vi "MEMR-Initialize Stimuli.vi"(0 "Data folder":path, 5 "Params":T31, 7 "AO in":T1 {"noiseChan"."Filter"."Stages"."IIR Filter"."Forward Coefficients" format="%.4f"; "noiseChan"."Filter"."Stages"."IIR Filter"."Reverse Coefficients" format="%.4f"}, 11 "error in (no error)":errorcluster) -> (8 "AO out":T1 {"noiseChan"."Filter"."Stages"."IIR Filter"."Forward Coefficients" format="%.4f"; "noiseChan"."Filter"."Stages"."IIR Filter"."Reverse Coefficients" format="%.4f"}, 15 "error out":errorcluster)   [LabVIEW 2020]
uses:
  Typedefs/MEMR-Params.ctl
  Typedefs/MEMR-Probe.ctl
  Typedefs/MEMR-Elicitor.ctl
  Human Studies/SFM Frontend/LV Source/Typedefs/HSTS-Transducer.ctl
  Typedefs/MEMR-Sequence.ctl
  Typedefs/MEMR-Analysis.ctl
  Typedefs/MEMR-Timing.ctl
  Typedefs/MEMR-AO Data.ctl
  Signal Synthesis VIs/3rd Generation/XControls/Stimulus Channel (G3)/Full Stimulus Channel Data.ctl
  Signal Synthesis VIs/3rd Generation/XControls/Waveform XControls/Waveform (G3)/Waveform Data.ctl
  Signal Synthesis VIs/3rd Generation/Waveform VIs/Waveform Enum (V3).ctl
  Signal Synthesis VIs/3rd Generation/XControls/Waveform XControls/Tone (G3)/Tone.Properties.ctl
  Signal Synthesis VIs/Waveform VIs/Pulse Train VIs/Pulse Train Params.ctl
  Signal Synthesis VIs/Waveform VIs/Pulse Train VIs/Pulse Polarity.ctl
  Signal Synthesis VIs/Waveform VIs/Pulse Train VIs/PT-Continuous State.ctl
  Signal Synthesis VIs/3rd Generation/Waveform VIs/Noise VIs/Noise (G3).ctl
  Signal Synthesis VIs/3rd Generation/Waveform VIs/Noise VIs/Noise (G3).Properties.ctl
  Signal Synthesis VIs/3rd Generation/Waveform VIs/Noise VIs/Noise (G3).Data.ctl
  Signal Synthesis VIs/Waveform VIs/File VIs/StimFile-Params.ctl
  Signal Synthesis VIs/Waveform VIs/FM Sweep VIs/FM Sweep Params.ctl
  Signal Synthesis VIs/Waveform VIs/Chirp Train VIs/Chirp Train.ctl
  Signal Synthesis VIs/Waveform VIs/Chirp Train VIs/Chirp Train Params.ctl
  Signal Synthesis VIs/Waveform VIs/Complex Tone VIs/CT-Params.ctl
  Signal Synthesis VIs/Waveform VIs/Complex Tone VIs/CT-Phase Enum.ctl
  Signal Synthesis VIs/Waveform VIs/Complex Tone VIs/CT-Runtime Data.ctl
  Signal Synthesis VIs/3rd Generation/XControls/Waveform XControls/FM Tone/Data.ctl
  Signal Synthesis VIs/3rd Generation/XControls/Waveform XControls/Vowel/Vowel.Properties.ctl
  Signal Synthesis VIs/3rd Generation/Waveform VIs/Ramp VIs/Ramp.Properties.ctl
  Signal Synthesis VIs/3rd Generation/XControls/Filter (G3)/Filter Data.ctl
  Signal Synthesis VIs/3rd Generation/XControls/Filter (G3)/Filter Type.ctl
  Signal Synthesis VIs/Filter VIs/Filter-Bandwidth Units.ctl
  Signal Synthesis VIs/Controls/Burst XCtl/Burst Data.ctl
  Signal Synthesis VIs/3rd Generation/XControls/Level (G3)/Level Data.ctl
  Signal Synthesis VIs/3rd Generation/XControls/Level (G3)/Level Units (G3).ctl
  Signal Synthesis VIs/3rd Generation/XControls/Advanced Options (G3)/Advanced Options (G3).ctl
  Signal Synthesis VIs/Modulation VIs/SAM VIs/SAM Params.ctl
  Signal Synthesis VIs/3rd Generation/Typedefs/Destination.ctl
  PXI DAQ VIs/DAQ Engine VIs/PXI Globals.vi
  Utility VIs/Math VIs/LinSpace (start-stop-step).vi
  Utility VIs/Math VIs/dB to Linear (1D).vi
  Signal Synthesis VIs/3rd Generation/XControls/Waveform XControls/Tone (G3)/Tone (G3).xctl
  Signal Synthesis VIs/3rd Generation/XControls/Waveform XControls/FM Tone/FM Tone.xctl
  Signal Synthesis VIs/3rd Generation/XControls/Waveform XControls/Vowel/Vowel.xctl
  Signal Synthesis VIs/3rd Generation/XControls/Waveform XControls/Waveform (G3)/Waveform (G3).xctl
  Signal Synthesis VIs/3rd Generation/XControls/Filter (G3)/Filter (G3).xctl
  Signal Synthesis VIs/Controls/Burst XCtl/Burst Control.xctl
  Signal Synthesis VIs/3rd Generation/XControls/Level (G3)/Level (G3).xctl
  Signal Synthesis VIs/3rd Generation/XControls/Advanced Options (G3)/Advanced Options (G3).xctl
  Signal Synthesis VIs/3rd Generation/XControls/Stimulus Channel (G3)/Stimulus Channel (G3).xctl
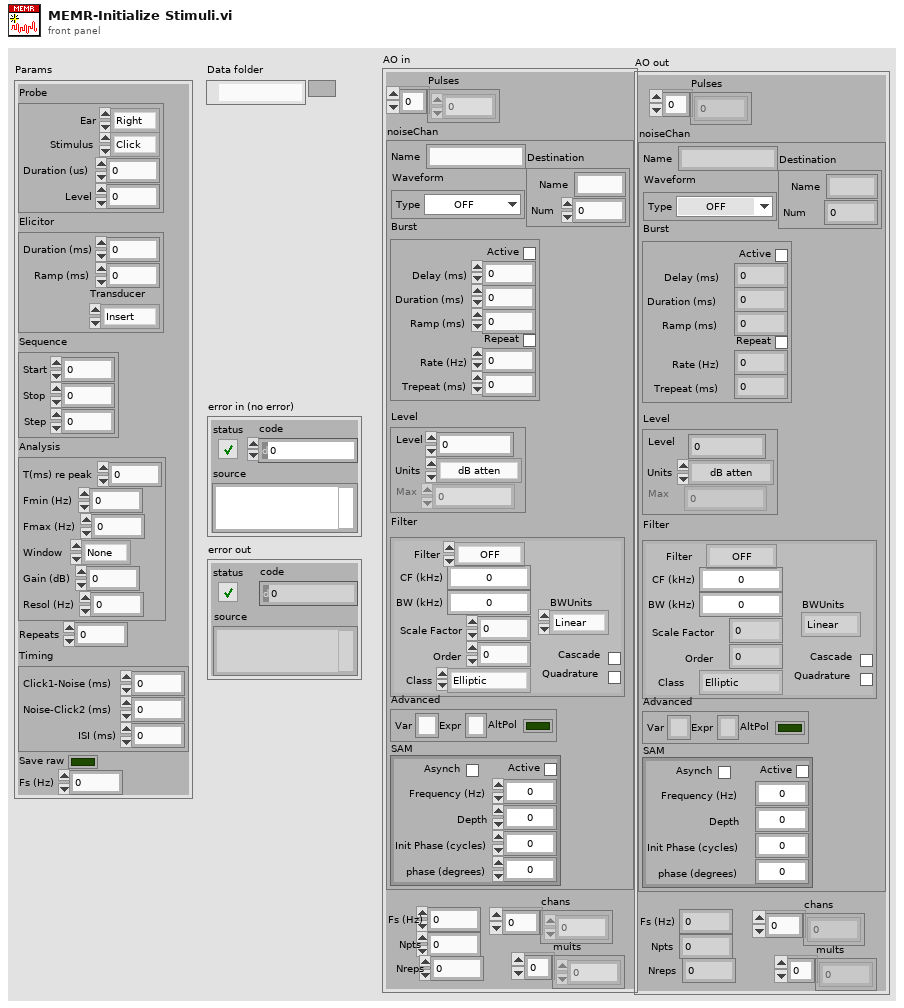
[diagram p1: front panel]
types:
  T1 = typedef "MEMR-AO Data.ctl" = cluster{"Pulses":dbl[], "noiseChan":T2, "Fs (Hz)":dbl, "Npts":i32, "mults":dbl[], "chans":i32[], "Nreps":i32}
  T2 = typedef "Stimulus Channel (G3).xctl/Full Stimulus Channel Data.ctl" = cluster{"Waveform":T3, "Filter":T22, "Burst":T25, "Level":T26, "Name":string, "Advanced":T28, "SAM":T29, "Destination":T30}
  T3 = typedef "Waveform (G3).xctl/Waveform Data.ctl" = cluster{"Type":T4, "Tone":T5, "Pulse Train":T6, "Noise":T9, "File":T12, "FMSweep":T13, "Chirp Train":T14, "Complex Tone":cluster{"Params":T16, "Data":T18}, "FM":T19, "Vowel":T20, "Ramp":T21}
  T4 = typedef "Waveform Enum (V3).ctl" = enum16{"OFF", "Tone", "Noise", "Pulse Train", "File", "FM Sweep", "Chirp Train", "Complex Tone", "FM Tone", "Vowel", "Ramp"}
  T5 = typedef "Tone (G3).xctl/Tone.Properties.ctl" = cluster{"Frequency (kHz)":dbl, "Phase (cycles)":dbl, "Random phase":bool}
  T6 = typedef "Pulse Train Params.ctl" = cluster{"Pulse width (us)":dbl, "Pulse rate (Hz)":dbl, "Gap (ms)":dbl, "Polarity":T7, "PT State":T8, "Asynch":bool}
  T7 = typedef "Pulse Polarity.ctl" = enum16{"POS", "NEG", "POS-NEG", "NEG-POS"}
  T8 = typedef "PT-Continuous State.ctl" = cluster{"Template":dbl[], "Nperiod":i32, "Index":i32, "Pulse Rate (Hz)":dbl, "Phase (cycles)":dbl, "Noff":i32}
  T9 = typedef "Noise (G3).ctl" = cluster{"Properties":T10, "Data":T11}
  T10 = typedef "Noise (G3).Properties.ctl" = cluster{"InvFilt":bool, "Aweight":bool, "Seed":i32, "Tokens":i32, "Brickwall":bool}
  T11 = typedef "Noise (G3).Data.ctl" = cluster{"TokenNum":i32}
  T12 = typedef "StimFile-Params.ctl" = cluster{"Filename":path, "Signal":dbl[], "Channel":i32, "stream":bool, "offset":i32, "nreps":i32, "loops":i32, "Randomize":bool, "order":i32[], "Seed":i32, "Tokens":i32}
  T13 = typedef "FM Sweep Params.ctl" = cluster{"Rate (oct/s)":dbl, "Fmin (Hz)":dbl, "Fmax (Hz)":dbl, "Ramp (ms)":dbl, "Linear":bool}
  T14 = typedef "Chirp Train.ctl" = cluster{"Params":T15, "Data":cluster{"WF":dbl[]}}
  T15 = typedef "Chirp Train Params.ctl" = cluster{"Fmin (kHz)":dbl, "Fmax (kHz)":dbl, "Compensate":bool, "Duration (ms)":dbl}
  T16 = typedef "CT-Params.ctl" = cluster{"F0 (Hz)":dbl, "Band":cluster{"Flow (Hz)":dbl, "Fhigh (Hz)":dbl}, "Phase":T17, "Min F0 (Hz)":dbl, "Max F0 (Hz)":dbl, "ContinRandPhase":bool, "Max peak factor":dbl, "Max mod depth":dbl, "MinHarmNum":i32, "MaxHarmNum":i32, "Level Mode":enum16{"per component", "overall rms"}, "% jitter":dbl}
  T17 = typedef "CT-Phase Enum.ctl" = enum16{"Cosine", "Random", "Alternating"}
  T18 = typedef "CT-Runtime Data.ctl" = cluster{"Ncomp":i32, "MinHarm":i32, "Phase":dbl[], "Amplitude":dbl[], "Npts/frame":i32, "Last F0":dbl, "Fmin":dbl, "Fmax":dbl, "Lslope":dbl, "randphase":bool, "overall rms":bool, "fmult":dbl[], "jittered":bool}
  T19 = typedef "FM Tone.xctl/Data.ctl" = cluster{"Carrier (kHz)":dbl, "ModRate (Hz)":dbl, "Depth (Hz)":dbl, "Phase (cycles)":dbl}
  T20 = typedef "Vowel.xctl/Vowel.Properties.ctl" = cluster{"Freqs":string, "Set level":enum16{"Total", "Per component"}, "Freq":dbl[], "weights":dbl[]}
  T21 = typedef "Ramp.Properties.ctl" = cluster{"Duration (ms)":dbl}
  T22 = typedef "Filter (G3).xctl/Filter Data.ctl" = cluster{"Type":T23, "CF (kHz)":dbl, "BW (kHz)":dbl, "Cascade":bool, "Quadrature":bool, "Scale Factor":dbl, "Stages":cluster{"IIR Filter":cluster{"filter structure":enum32{"IIR 2nd Order", "IIR 4th Order"}, "Reverse Coefficients":dbl[], "Forward Coefficients":dbl[]}, "State":dbl[]}[], "Class":enum16{"Elliptic", "Butterworth"}, "Order":i32, "BWUnits":T24}
  T23 = typedef "Filter (G3).xctl/Filter Type.ctl" = enum16{"OFF", "Lowpass", "Highpass", "Bandpass", "Bandstop"}
  T24 = typedef "Filter-Bandwidth Units.ctl" = enum16{"Linear", "Octaves", "Min-Max"}
  T25 = typedef "Burst Control.xctl/Burst Data.ctl" = cluster{"Active":bool, "Delay (ms)":dbl, "Duration (ms)":dbl, "Ramp (ms)":dbl, "Rate (Hz)":dbl, "Trepeat (ms)":dbl, "Repeat":bool}
  T26 = typedef "Level (G3).xctl/Level Data.ctl" = cluster{"Level":dbl, "Units":T27, "Max":dbl, "Data":cluster{"Multiplier":dbl, "Cal File":path, "Cal":cluster{"Freq (Hz)":dbl[], "Mag (dB SPL)":dbl[], "Phase (deg)":dbl[]}, "audiogram":path}}
  T27 = typedef "Level (G3).xctl/Level Units (G3).ctl" = enum16{"dB atten", "dB SPL", "dB re 1 Vrms", "dB V/Hz½", "mW", "dB HL", "Volts", "dB mW"}
  T28 = typedef "Advanced Options (G3).xctl/Advanced Options (G3).ctl" = cluster{"AltPol":bool, "Var":string, "Expr":string}
  T29 = typedef "SAM Params.ctl" = cluster{"Active":bool, "Frequency (Hz)":dbl, "Depth":dbl, "Init Phase (cycles)":dbl, "phase (degrees)":dbl, "Asynch":bool}
  T30 = typedef "Destination.ctl" = cluster{"Name":string, "Num":i32}
  T31 = typedef "MEMR-Params.ctl" = cluster{"Probe":T32, "Elicitor":T33, "Sequence":T35, "Analysis":T36, "Repeats":i32, "Timing":T37, "Save raw":bool, "Fs (Hz)":dbl}
  T32 = typedef "MEMR-Probe.ctl" = cluster{"Ear":enum16{"Right", "Left"}, "Stimulus":enum16{"Click", "Chirp"}, "Duration (us)":dbl, "Level":dbl}
  T33 = typedef "MEMR-Elicitor.ctl" = cluster{"Duration (ms)":dbl, "Ramp (ms)":dbl, "Transducer":T34}
  T34 = typedef "HSTS-Transducer.ctl" = enum16{"Insert", "TDH-39", "HD300", "ER-10X"}
  T35 = typedef "MEMR-Sequence.ctl" = cluster{"Start":dbl, "Stop":dbl, "Step":dbl}
  T36 = typedef "MEMR-Analysis.ctl" = cluster{"T(ms) re peak":dbl, "Fmin (Hz)":dbl, "Fmax (Hz)":dbl, "Window":enum16{"None", "Hanning", "Hamming"}, "Gain (dB)":dbl, "Resol (Hz)":dbl}
  T37 = typedef "MEMR-Timing.ctl" = cluster{"Click1-Noise (ms)":dbl, "Noise-Click2 (ms)":dbl, "ISI (ms)":dbl}
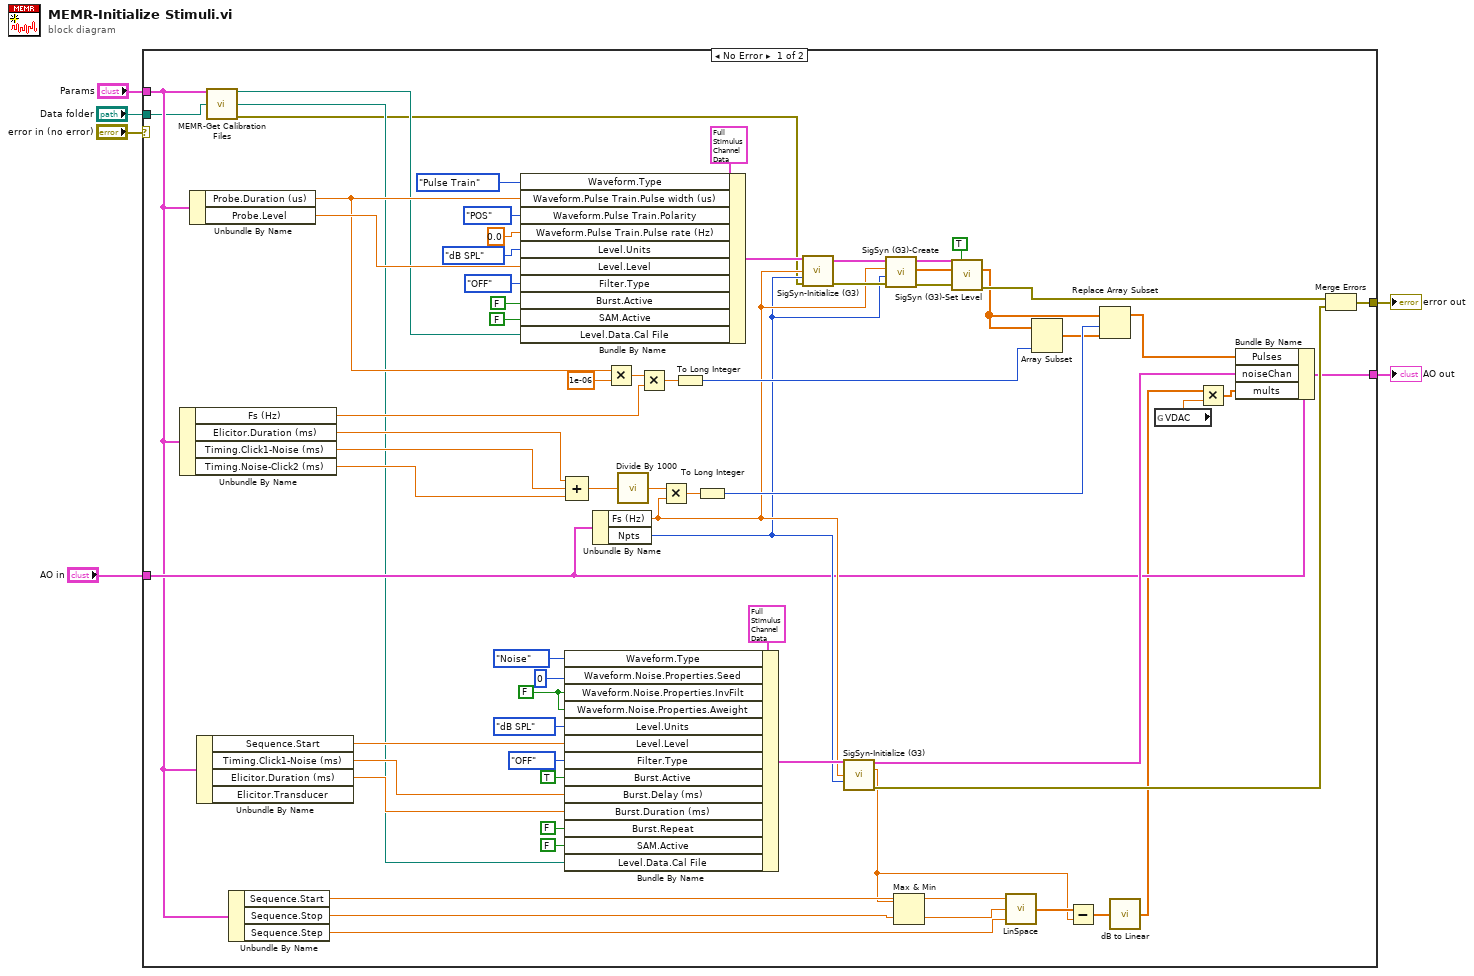
[diagram p0: block diagram]
diagram:
  n1 = case shown="No Error" "error in (no error)" {
    selector: "error in (no error)" -> [_ w75]
    tunnel: "Data folder" -> [w8 _]
    tunnel: [w37 w75] -> w4
    tunnel: "Params" -> [w12 _]
    tunnel: [w25 _] -> w2
    tunnel: "AO in" -> [w22 _]
    frame No Error {
      w48 = FALSE ("Waveform.Noise.Properties.InvFilt")
      n2 = Unbundle By Name(w12) -> ("Fs (Hz)"=w34:dbl, "Elicitor.Duration (ms)"=w62:dbl, "Timing.Click1-Noise (ms)"=w61:dbl, "Timing.Noise-Click2 (ms)"=w60:dbl)
      n3 = Unbundle By Name(w12) -> ("Probe.Duration (us)"=w56:dbl, "Probe.Level"=w69:dbl)
      n4 = Unbundle By Name(w12) -> ("Sequence.Start"=w46:dbl, "Timing.Click1-Noise (ms)"=w43:dbl, "Elicitor.Duration (ms)"=w42:dbl)  [unwired: 1 out]
      n5 = call "MEMR-Get Calibration Files.vi"("Params"=w12, "Data Folder"=w8) -> ("Probe"=w11:path, "Elicitor"=w10:path, "error out"=w9:errorcluster)  [unwired: 11 in]
      n6 = Unbundle By Name(w12) -> ("Sequence.Start"=w32:dbl, "Sequence.Stop"=w30:dbl, "Sequence.Step"=w31:dbl)
      n7 = Bundle By Name(cluster=T2 {"Waveform"={"Type"=enum."Tone", "Tone"={"Frequency (kHz)"=0.0, "Phase (cycles)"=0.0, "Random phase"=FALSE}, "Pulse Train"={"Pulse width (us)"=0.0, "Pulse rate (Hz)"=0.0, "Gap (ms)"=0.0, "Polarity"=enum."POS", "PT State"={"Template"=[], "Nperiod"=0, "Index"=0, "Pulse Rate (Hz)"=0.0, "Phase (cycles)"=0.0, "Noff"=0}, "Asynch"=FALSE}, "Noise"={"Properties"={"InvFilt"=FALSE, "Aweight"=FALSE, "Seed"=0, "Tokens"=0, "Brickwall"=FALSE}, "Data"={"TokenNum"=0}}, "File"={"Filename"=path "", "Signal"=[], "Channel"=0, "stream"=FALSE, "offset"=0, "nreps"=0, "loops"=0, "Randomize"=FALSE, "order"=[], "Seed"=0, "Tokens"=0}, "FMSweep"={"Rate (oct/s)"=0.0, "Fmin (Hz)"=0.0, "Fmax (Hz)"=0.0, "Ramp (ms)"=0.0, "Linear"=FALSE}, "Chirp Train"={"Params"={"Fmin (kHz)"=4.0, "Fmax (kHz)"=64.0, "Compensate"=FALSE, "Duration (ms)"=2.0}, "Data"={"WF"=[]}}, "Complex Tone"={"Params"={"F0 (Hz)"=0.0, "Band"={"Flow (Hz)"=0.0, "Fhigh (Hz)"=0.0}, "Phase"=enum."Cosine", "Min F0 (Hz)"=0.0, "Max F0 (Hz)"=0.0, "ContinRandPhase"=FALSE, "Max peak factor"=inf, "Max mod depth"=2.0, "MinHarmNum"=0, "MaxHarmNum"=0, "Level Mode"=enum."per component", "% jitter"=0.0}, "Data"={"Ncomp"=0, "MinHarm"=0, "Phase"=[], "Amplitude"=[], "Npts/frame"=0, "Last F0"=0.0, "Fmin"=0.0, "Fmax"=0.0, "Lslope"=0.0, "randphase"=FALSE, "overall rms"=FALSE, "fmult"=[], "jittered"=FALSE}}, "FM"={"Carrier (kHz)"=0.0, "ModRate (Hz)"=0.0, "Depth (Hz)"=0.0, "Phase (cycles)"=0.0}, "Vowel"={"Freqs"="", "Set level"=enum."Total", "Freq"=[], "weights"=[]}, "Ramp"={"Duration (ms)"=0.0}}, "Filter"={"Type"=enum."Lowpass", "CF (kHz)"=0.0, "BW (kHz)"=0.0, "Cascade"=FALSE, "Quadrature"=FALSE, "Scale Factor"=0.0, "Stages"=[], "Class"=enum."Elliptic", "Order"=0, "BWUnits"=enum."Linear"}, "Burst"={"Active"=FALSE, "Delay (ms)"=0.0, "Duration (ms)"=0.0, "Ramp (ms)"=0.0, "Rate (Hz)"=0.0, "Trepeat (ms)"=0.0, "Repeat"=FALSE}, "Level"={"Level"=0.0, "Units"=enum."dB atten", "Max"=0.0, "Data"={"Multiplier"=0.0, "Cal File"=path "", "Cal"={"Freq (Hz)"=[], "Mag (dB SPL)"=[], "Phase (deg)"=[]}, "audiogram"=path ""}}, "Name"="", "Advanced"={"AltPol"=FALSE, "Var"="", "Expr"=""}, "SAM"={"Active"=FALSE, "Frequency (Hz)"=0.0, "Depth"=0.0, "Init Phase (cycles)"=0.0, "phase (degrees)"=0.0, "Asynch"=FALSE}, "Destination"={"Name"="", "Num"=0}} ("Stimulus"), "Waveform.Type"=Waveform_Enum_(V3)."Pulse Train", "Waveform.Pulse Train.Pulse width (us)"=w56, "Waveform.Pulse Train.Polarity"=Pulse_Polarity."POS", "Waveform.Pulse Train.Pulse rate (Hz)"=0.0, "Level.Units"=Level_Units_(G3)."dB SPL", "Level.Level"=w69, "Filter.Type"=Filter_Type."OFF", "Burst.Active"=FALSE, "SAM.Active"=FALSE, "Level.Data.Cal File"=w11) -> (w65:T2)
      n8 = Bundle By Name(cluster=T2 {"Waveform"={"Type"=enum."Tone", "Tone"={"Frequency (kHz)"=0.0, "Phase (cycles)"=0.0, "Random phase"=FALSE}, "Pulse Train"={"Pulse width (us)"=0.0, "Pulse rate (Hz)"=0.0, "Gap (ms)"=0.0, "Polarity"=enum."POS", "PT State"={"Template"=[], "Nperiod"=0, "Index"=0, "Pulse Rate (Hz)"=0.0, "Phase (cycles)"=0.0, "Noff"=0}, "Asynch"=FALSE}, "Noise"={"Properties"={"InvFilt"=FALSE, "Aweight"=FALSE, "Seed"=0, "Tokens"=0, "Brickwall"=FALSE}, "Data"={"TokenNum"=0}}, "File"={"Filename"=path "", "Signal"=[], "Channel"=0, "stream"=FALSE, "offset"=0, "nreps"=0, "loops"=0, "Randomize"=FALSE, "order"=[], "Seed"=0, "Tokens"=0}, "FMSweep"={"Rate (oct/s)"=0.0, "Fmin (Hz)"=0.0, "Fmax (Hz)"=0.0, "Ramp (ms)"=0.0, "Linear"=FALSE}, "Chirp Train"={"Params"={"Fmin (kHz)"=4.0, "Fmax (kHz)"=64.0, "Compensate"=FALSE, "Duration (ms)"=2.0}, "Data"={"WF"=[]}}, "Complex Tone"={"Params"={"F0 (Hz)"=0.0, "Band"={"Flow (Hz)"=0.0, "Fhigh (Hz)"=0.0}, "Phase"=enum."Cosine", "Min F0 (Hz)"=0.0, "Max F0 (Hz)"=0.0, "ContinRandPhase"=FALSE, "Max peak factor"=inf, "Max mod depth"=2.0, "MinHarmNum"=0, "MaxHarmNum"=0, "Level Mode"=enum."per component", "% jitter"=0.0}, "Data"={"Ncomp"=0, "MinHarm"=0, "Phase"=[], "Amplitude"=[], "Npts/frame"=0, "Last F0"=0.0, "Fmin"=0.0, "Fmax"=0.0, "Lslope"=0.0, "randphase"=FALSE, "overall rms"=FALSE, "fmult"=[], "jittered"=FALSE}}, "FM"={"Carrier (kHz)"=0.0, "ModRate (Hz)"=0.0, "Depth (Hz)"=0.0, "Phase (cycles)"=0.0}, "Vowel"={"Freqs"="", "Set level"=enum."Total", "Freq"=[], "weights"=[]}, "Ramp"={"Duration (ms)"=0.0}}, "Filter"={"Type"=enum."Lowpass", "CF (kHz)"=0.0, "BW (kHz)"=0.0, "Cascade"=FALSE, "Quadrature"=FALSE, "Scale Factor"=0.0, "Stages"=[], "Class"=enum."Elliptic", "Order"=0, "BWUnits"=enum."Linear"}, "Burst"={"Active"=FALSE, "Delay (ms)"=0.0, "Duration (ms)"=0.0, "Ramp (ms)"=0.0, "Rate (Hz)"=0.0, "Trepeat (ms)"=0.0, "Repeat"=FALSE}, "Level"={"Level"=0.0, "Units"=enum."dB atten", "Max"=0.0, "Data"={"Multiplier"=0.0, "Cal File"=path "", "Cal"={"Freq (Hz)"=[], "Mag (dB SPL)"=[], "Phase (deg)"=[]}, "audiogram"=path ""}}, "Name"="", "Advanced"={"AltPol"=FALSE, "Var"="", "Expr"=""}, "SAM"={"Active"=FALSE, "Frequency (Hz)"=0.0, "Depth"=0.0, "Init Phase (cycles)"=0.0, "phase (degrees)"=0.0, "Asynch"=FALSE}, "Destination"={"Name"="", "Num"=0}} ("Stimulus"), "Waveform.Type"=Waveform_Enum_(V3)."Noise", "Waveform.Noise.Properties.Seed"=0, "Waveform.Noise.Properties.InvFilt"=w48, "Waveform.Noise.Properties.Aweight"=w48, "Level.Units"=Level_Units_(G3)."dB SPL", "Level.Level"=w46, "Filter.Type"=Filter_Type."OFF", "Burst.Active"=TRUE, "Burst.Delay (ms)"=w43, "Burst.Duration (ms)"=w42, "Burst.Repeat"=FALSE, "SAM.Active"=FALSE, "Level.Data.Cal File"=w10) -> (w39:T2)
      n9 = Compound Arithmetic op=ADD(w62, w61, w60) -> (w57:dbl)
      n10 = Unbundle By Name(w22) -> ("Fs (Hz)"=w24:dbl, "Npts"=w23:i32)
      n11 = Multiply(x=w56, y=1e-06) -> (x*y=w53:dbl)
      n12 = call "Divide By 1000.vi"("X"=w57) -> ("X/1000"=w59:dbl)
      n13 = Multiply(x=w53, y=w34) -> (x*y=w54:dbl)
      n14 = Multiply(x=w59, y=w24) -> (x*y=w58:dbl)
      n15 = To Long Integer(number=w54) -> (32bit integer=w33:i32)
      n16 = To Long Integer(number=w58) -> (32bit integer=w52:i32)
      n17 = call "SigSyn-Initialize (G3).vi"("Stimulus Channel"=w65, "Sampling rate (Hz)"=w24, "Npts"=w23, "error in (no error)"=w9) -> ("Stimulus Channel out"=w63:T2, "error out"=w64:errorcluster)  [unwired: 9 in, 1 out]
      n18 = call "SigSyn-Initialize (G3).vi"("Stimulus Channel"=w39, "Sampling rate (Hz)"=w24, "Npts"=w23) -> ("Stimulus Channel out"=w35:T2, "Max Level"=w27:dbl, "error out"=w38:errorcluster)  [unwired: 10 in]
      n19 = call "SigSyn (G3)-Create.vi"("error in (no error)"=w64, "Npts"=w23, "Sampling Rate (Hz)"=w24, "Stimulus Channel"=w63) -> ("error out"=w16:errorcluster, "Waveform"=w17:dbl[], "Stimulus Channel out"=w18:T2)  [unwired: 4 in, 1 out]
      n20 = Max & Min(x=w27, y=w30) -> (min(x,y)=w29:dbl)  [unwired: 1 out]
      n21 = call "SigSyn (G3)-Set Level.vi"("StimChans In"=w18, "Apply multiplier? (F)"=TRUE, "Waveform in"=w17, "error in (no error)"=w16) -> ("Waveform out"=w14:dbl[], "error out"=w15:errorcluster)  [unwired: 7 in, 3 out]
      n22 = call-poly "LinSpace.vi"("Step"=w31, "Stop"=w29, "Start"=w32) -> ("Array"=w28:dbl[])  [unwired: 1 in, 1 out]
      n23 = Array Subset(array=w14, length=w33) -> (w7:dbl[])  [unwired: 1 in]
      n24 = Subtract(x=w28, y=w27) -> (x-y=w26:dbl[])
      n25 = Replace Array Subset(array=w14, new element=w7, index=w52) -> (w36:dbl[])
      n26 = call-poly "dB to Linear.vi"("dB"=w26) -> ("linear"=w21:dbl[])
      n27 = global read "PXI Globals.vi" "VDAC"() -> (w19:dbl)
      n28 = Multiply(x=w21, y=w19) -> (x*y=w20:dbl[])
      n29 = Bundle By Name(cluster=w22, "Pulses"=w36, "noiseChan"=w35, "mults"=w20) -> (w25:T1)
      n30 = Merge Errors(w15, w38) -> (w37:errorcluster)
    }
    frame Error {
    }
  }
  "error out" <- w4
  "AO out" <- w2
